vi "PCP 24bit pulse counter convert to signed.vi"(10 "24 bit puls counter input":i32) -> (2 "signed pulse counter output":i32)   [LabVIEW 2011]
doc: "This VI detects if the value from a pulse counter is negative or positive. It will split the range of a 24 bit pulse counter in two."
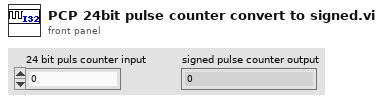
[diagram p1: front panel]
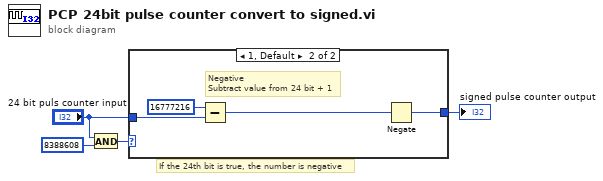
[diagram p0: block diagram]
diagram:
  # "If the 24th bit is true, the number is negative"
  n1 = And(x="24 bit puls counter input", y=8388608) -> (x .and. y?=w4:i32)
  n2 = case shown="1, Default" w4 {
    tunnel: "24 bit puls counter input" -> [w5 w8]
    tunnel: [w5 w9] -> w2
    frame 0 {
      # "Positive\nDo nothing"
    }
    frame 1, Default {
      # "Negative\nSubtract value from 24 bit + 1"
      n3 = Subtract(x=16777216 ("y"), y=w8) -> (x-y=w7:i32)
      n4 = Negate(x=w7) -> (-x=w9:i32)
    }
  }
  "signed pulse counter output" <- w2
